vi "LV RT Doc - Instantiate with Path.vi"(0 "LV Doc Path":path, 11 "error in (no error)":errorcluster) -> (4 "LV RT":refnum<class "LV RT.lvclass">, 15 "error out":errorcluster)   [LabVIEW 2019, in "LV RT.lvclass"]
uses:
  LV RT.lvclass
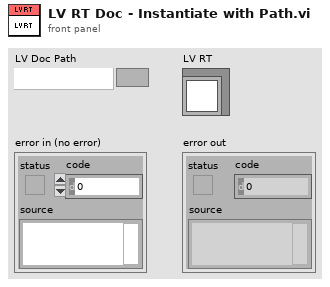
[diagram p1: front panel]
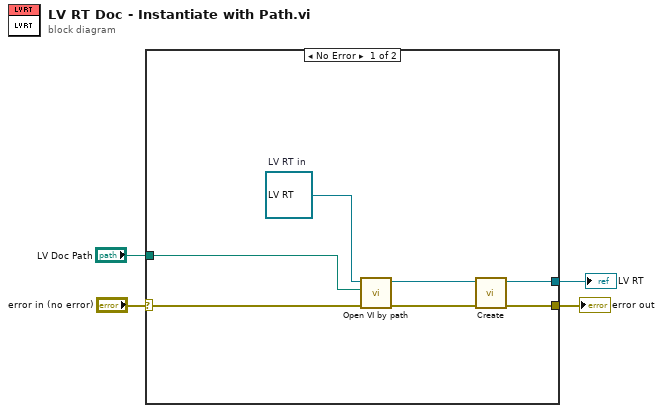
[diagram p0: block diagram]
diagram:
  n1 = case shown="No Error" "error in (no error)" {
    selector: "error in (no error)" -> [w7 w12]
    tunnel: [w10 w12] -> w3
    tunnel: "LV Doc Path" -> [w8 _]
    tunnel: [w11 _] -> w1
    frame No Error {
      w9 = refnum<class "LV RT.lvclass"> refnum  # LV RT in
      n2 = call "Open VI by path.vi"("error in (no error)"=w7, "vi path"=w8, "LV RT in"=w9) -> ("error out"=w6:errorcluster, "LV RT out"=w5:refnum<class "LV RT.lvclass">)  [unwired: 7 in]
      n3 = call-dynamic "Create.vi"("error in (no error)"=w6, "Document in"=w5) -> ("error out"=w10:errorcluster, "Document out"=w11:refnum<class "LV RT.lvclass">)  [unwired: 8 in]
    }
    frame Error {
    }
  }
  "error out" <- w3
  "LV RT" <- w1
